vi "SSC Digital Clock Generator Generate Clock.vi"(0 "Digital SSC in":T1[](array[typedef]), 2 "select digital function?":bool=TRUE caption="select digital function? (T)", 5 "Frequency (Hz)":dbl=1000000.0 format="%#_6p", 11 "error in":errorcluster) -> (4 "Digital SSC out":T1[](array[typedef]), 15 "error out":errorcluster)   [LabVIEW 2019]
doc: "Configures clock generator frequency and initiates clock generation on the device(s) connected to the specified pin(s) and pin group(s)."
uses:
  SSC Digital.ctl
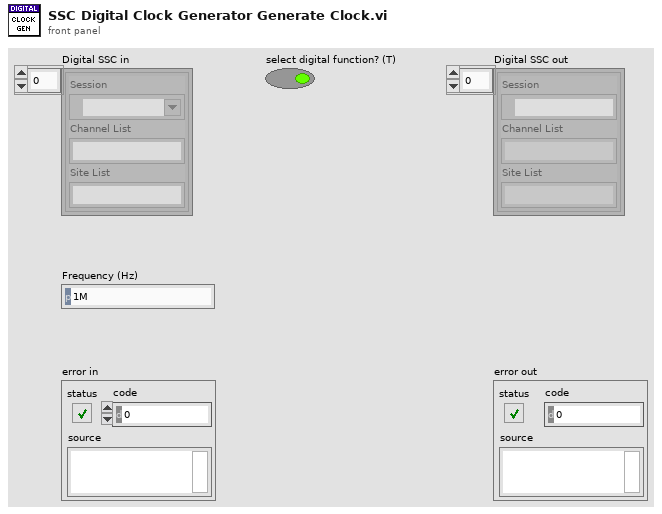
[diagram p1: front panel]
types:
  T1 = typedef "SSC Digital.ctl" = cluster{"Session":refnum<k15>, "Channel List":string, "Site List":string}
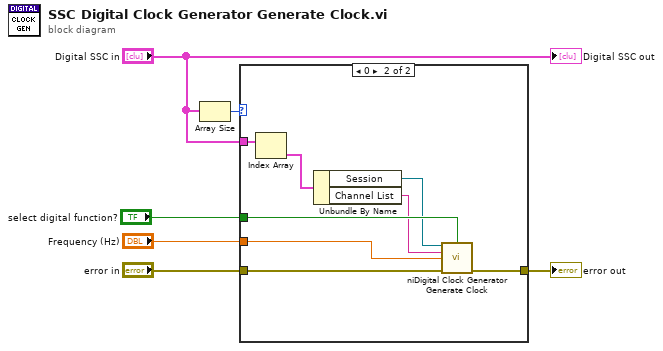
[diagram p0: block diagram]
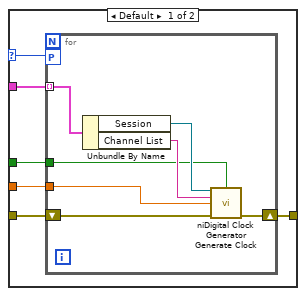
[diagram p2: hidden frame]
diagram:
  n1 = Array Size(array="Digital SSC in") -> (size(s)=w2:i32)
  n2 = case shown="0" w2 {
    selector: w2 -> [w8 _]
    tunnel: "Frequency (Hz)" -> [w12 w27]
    tunnel: "error in" -> [w11 w26]
    tunnel: [w10 w25] -> w4
    tunnel: "select digital function?" -> [w9 w24]
    tunnel: "Digital SSC in" -> [w7 w23]
    frame Default {
      n3 = for {
        workers-P: w8 -> [_]
        tunnel: w7 -> [w18] mode=indexing
        tunnel: w12 -> [w14]
        shift-right: [w15] -> w10
        shift-left: w11 -> [w19]
        tunnel: w9 -> [w13]
        n4 = Unbundle By Name(w18) -> ("Session"=w17:refnum<k15>, "Channel List"=w16:string)
        n5 = call <instrlib>:"niDigital Clock Generator Generate Clock.vi"("instrument handle"=w17, "select digital function? (T)"=w13, "channel list"=w16, "frequency (Hz)"=w14, "error in"=w19) -> ("error out"=w15:errorcluster)  [unwired: 9 in, 1 out]
      }
    }
    frame 0 {
      n6 = Index Array(array=w23) -> (element=w20:T1)  [unwired: 1 in]
      n7 = Unbundle By Name(w20) -> ("Session"=w22:refnum<k15>, "Channel List"=w21:string)
      n8 = call <instrlib>:"niDigital Clock Generator Generate Clock.vi"("instrument handle"=w22, "select digital function? (T)"=w24, "channel list"=w21, "frequency (Hz)"=w27, "error in"=w26) -> ("error out"=w25:errorcluster)  [unwired: 9 in, 1 out]
    }
  }
  "error out" <- w4
  "Digital SSC out" <- "Digital SSC in"
